vi "周期设置.vi"(7 "seconds since 1Jan1904":timestamp, 8 "质控启动日期":string(combo)="关闭", 9 "跨度核查时间":u16(ring)=6 items=["00H", "01H", "02H", "03H", "04H", "05H", "06H", "07H", "08H", "09H", "10H", "11H", "12H", "13H", "14H", "15H", "16H", "17H", "18H", "19H", "20H", "21H", "22H", "23H", "关闭"], 10 "零点核查时间":u16(ring)=2 items=["00H", "01H", "02H", "03H", "04H", "05H", "06H", "07H", "08H", "09H", "10H", "11H", "12H", "13H", "14H", "15H", "16H", "17H", "18H", "19H", "20H", "21H", "22H", "23H", "关闭"], 11 "运行模式":enum16{"维护模式", "常规模式", "应急模式", "质控模式"}(ring)) -> (1 "跨度核查启动命令":bool, 2 "零点核查启动命令":bool, 3 "水样测试启动命令":bool)   [LabVIEW 2016]
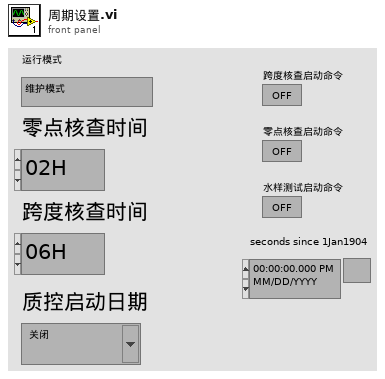
[diagram p1: front panel]
types:
  T1 = typedef "LVDateTimeRec.ctl" = cluster{"秒数的小数部分":dbl, "秒":i32, "分":i32, "时":i32, "日":i32, "月":i32, "年":i32, "天数（周）":i32, "天数（年）":i32, "DST":i32}
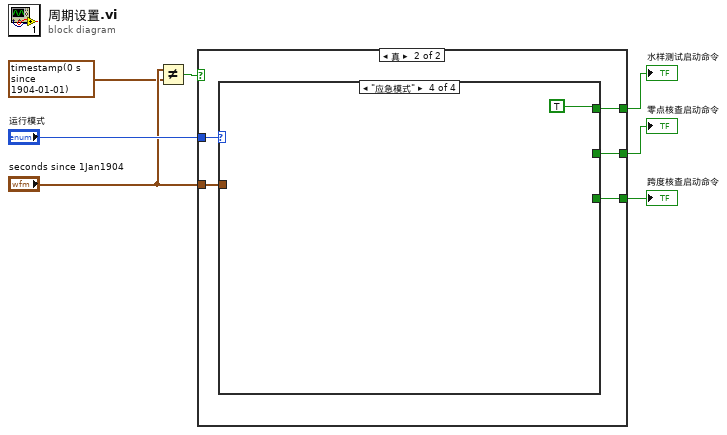
[diagram p0: block diagram]
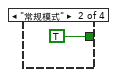
[diagram p4: hidden frame]
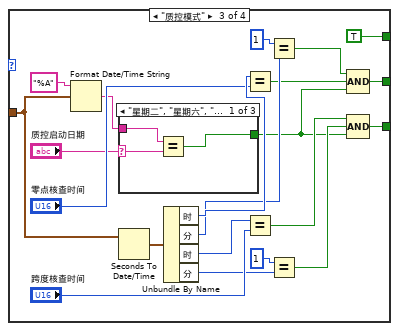
[diagram p5: hidden frame]
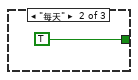
[diagram p6: hidden frame]
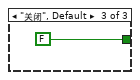
[diagram p7: hidden frame]
diagram:
  n1 = Not Equal?(x="seconds since 1Jan1904", y=timestamp(0 s since 1904-01-01)) -> (x != y?=w1:bool)
  n2 = case shown="真" w1 {
    tunnel: [_ w12] -> w7
    tunnel: [_ w11] -> w6
    tunnel: "运行模式" -> [_ w10]
    tunnel: [_ w9] -> w4
    tunnel: "seconds since 1Jan1904" -> [_ w8]
    frame False {
    }
    frame True {
      n3 = case shown="\"应急模式\"" w10 {
        tunnel: [_ _ w18 _] -> w12
        tunnel: [_ _ w17 _] -> w11
        tunnel: [_ TRUE TRUE TRUE] -> w9
        tunnel: w8 -> [_ _ w16 _]
        frame "维护模式", Default {
        }
        frame "常规模式" {
        }
        frame "质控模式" {
          n4 = Format Date/Time String(time format string (%c)="%A" ("时间格式字符串(%c)"), seconds (now)=w16) -> (date/time string=w20:string)  [unwired: 1 in]
          n5 = case shown="\"星期二\", \"星期六\", \"星期日\", \"星期三\", \"星期四\", \"星期五\", \"星期一\"" "质控启动日期" {
            selector: "质控启动日期" -> [w37 _ _]
            tunnel: [w36 TRUE FALSE] -> w22
            tunnel: w20 -> [w35 _ _]
            frame "星期二", "星期六", "星期日", "星期三", "星期四", "星期五", "星期一" {
              n6 = Equal?(x=w35, y=w37) -> (x = y?=w36:bool)
            }
            frame "每天" {
            }
            frame "关闭", Default {
            }
          }
          n7 = Seconds To Date/Time(time stamp (now)=w16) -> (date time rec=w34:T1)  [unwired: 1 in]
          n8 = Unbundle By Name(w34) -> ("时"=w33:i32, "分"=w31:i32, "时"=w27:i32, "分"=w26:i32)
          n9 = Equal?(x=w33, y="零点核查时间") -> (x = y?=w30:bool)
          n10 = Equal?(x=w27, y="跨度核查时间") -> (x = y?=w25:bool)
          n11 = Equal?(x=1, y=w31) -> (x = y?=w29:bool)
          n12 = Equal?(x=1, y=w26) -> (x = y?=w24:bool)
          n13 = Compound Arithmetic op=AND ("复合运算")(w29, w30, w22) -> (w17:bool)
          n14 = Compound Arithmetic op=AND ("复合运算")(w25, w24, w22) -> (w18:bool)
        }
        frame "应急模式" {
        }
      }
    }
  }
  "跨度核查启动命令" <- w7
  "零点核查启动命令" <- w6
  "水样测试启动命令" <- w4
